vi "Filtri acquisizioni in tabella prove NEW.vi"(11 "LINGUA":i32) -> ()   [LabVIEW 2019]
uses:
  Global percorso impostazioni.vi
  <vilib>/Utility/file.llb/Write Delimited Spreadsheet (string).vi
  <vilib>/Utility/file.llb/Read Delimited Spreadsheet (string).vi
panel:
  in  "APPLICA A TUTTE":bool
  in  "carica tabella":bool
  in  "TABELLA 2":u16(ring) items=["RES FREDDO RES METER", "RES FREDDO RESISTOMAT", "A VUOTO", "A CARICO", "TERMICA", "CMECC", "ROT BLOCC", "GENERICA", "ACQ RES TERMICA", "SCORTA 2", "SCORTA 3", "EQ.TERMICO", "COPPIA MAX", "I SPUNTO", "RES INIZ VUOTO", "RES FINE VUOTO", "RES INIZ CARICO", "RES FINE CARICO"]
  in  "TABELLA":u16(ring) items=["RES FREDDO RES METER", "RES FREDDO RESISTOMAT", "A VUOTO", "A CARICO", "TERMICA", "CMECC", "ROT BLOCC", "GENERICA", "ACQ RES TERMICA", "SCORTA 2", "SCORTA 3", "EQ.TERMICO", "COPPIA MAX", "I SPUNTO", "RES INIZ VUOTO", "RES FINE VUOTO", "RES INIZ CARICO", "RES FINE CARICO"]
  in  "ORDINE COLONNE":i32(listbox)
  in  "reinizializza":bool
  in  "Save Button":bool
  in  "stop":bool
  in  "Array":T1(array[cluster]) {"Medie RT" min=-1 max=100; "decimali" min=-1 max=5}
  in  "TIPO COLLEGAMENTO":u16(ring) items=["GRUPPO ELETTROGENO", "ALTERNATORE", "GENERICO", "MOTORE C.A.", "MOTORE EEX", "MOTORE C.C.", "POMPA", "TRASFORMATORE", "POMPA EEX"]
  # "VISIBILE?  SALVA?"
  # "seleziona\ntipo collegamento"
  # "nota: -1 sul campo \"decimali\" significa che\ni decimali della grandezza in questione\nnon vengono gestiti. Utilizzare -1 per le \ngrandezze che non sono valori numerici\nad esempio tempo[h:m:s]"
  # "CONDIZIONI OBBLIGATORIE:\n\nI seguenti campi:\n\n-Banco\n-Anno\n-Numero\n-N°tabella\n-Misura\n-Tipo prova\n-Progressivo Acq\n\ndevono avere decimali=0 ed\nessere salvati per tutte le prove\n\ni campI TESTO come\n\n-tempo[h:m:s]\n-Descrizione\n...\n\ndevono avere decimali=-1"
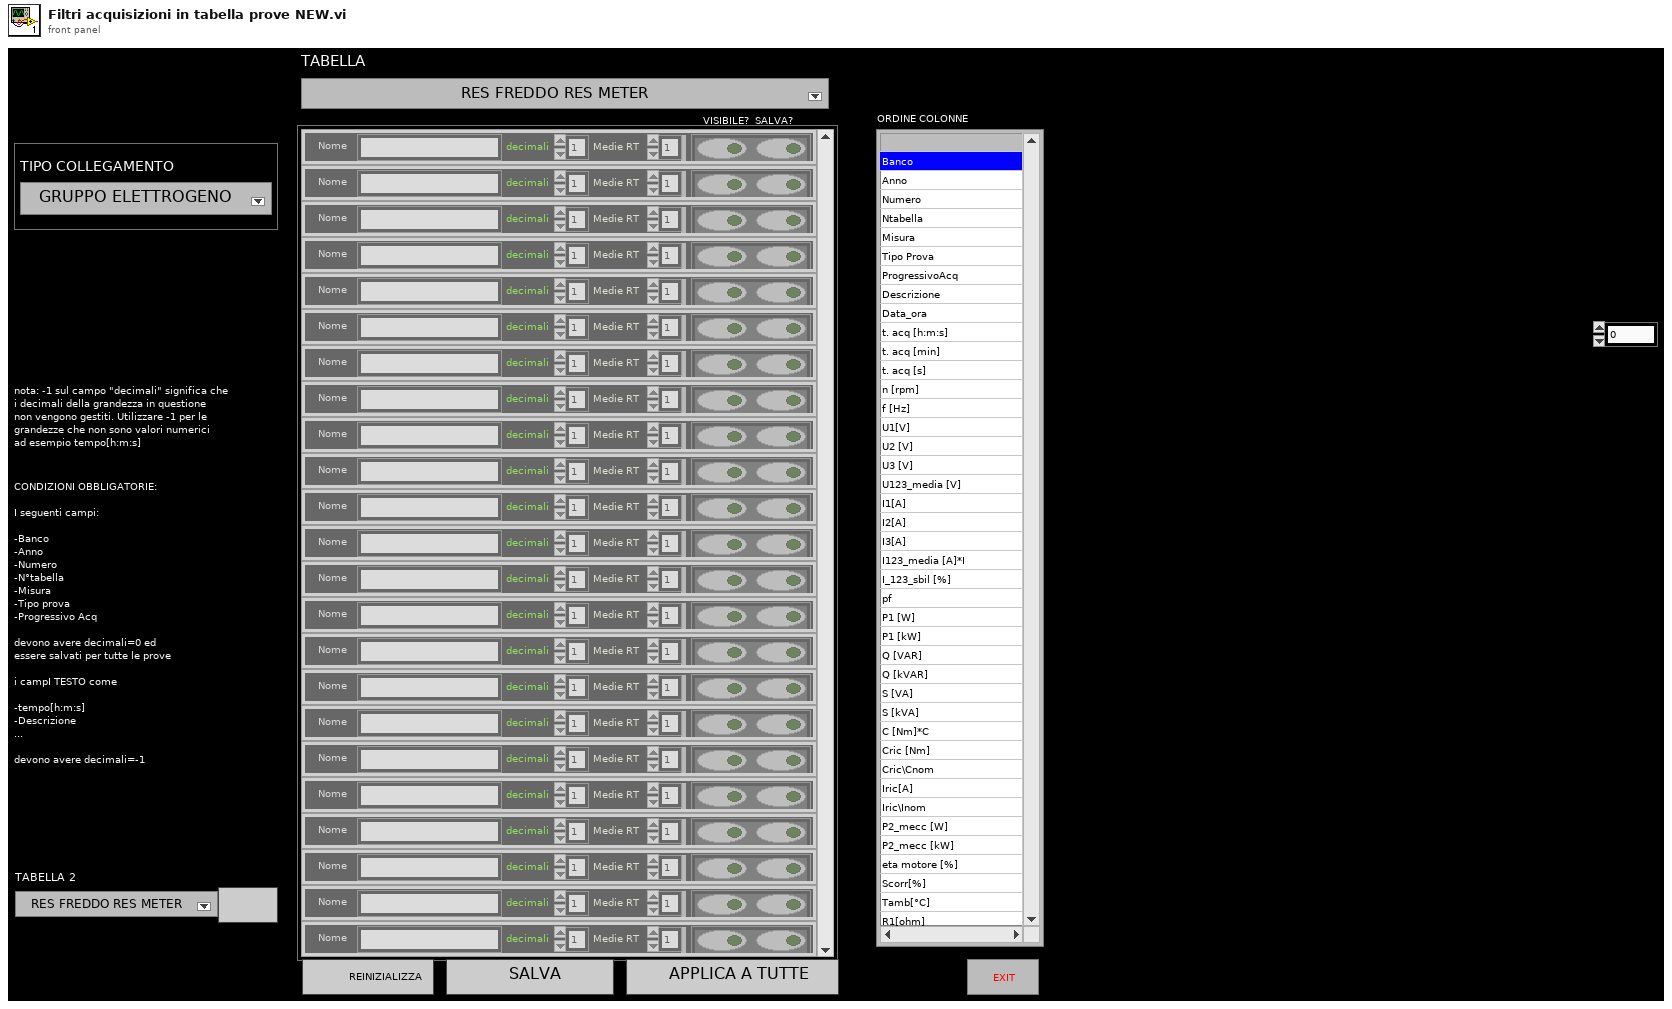
[diagram p1: front panel]
types:
  T1 = cluster{"Nome":string, "TAB":cluster{"Visibile ?":bool, "Salva?":bool}, "decimali":i8, "Medie RT":i8}[]
  T2 = cluster{"Nome":string, "TAB":cluster{"Visibile ?":bool, "Salva?":bool}, "decimali":i8, "Medie RT":i8}
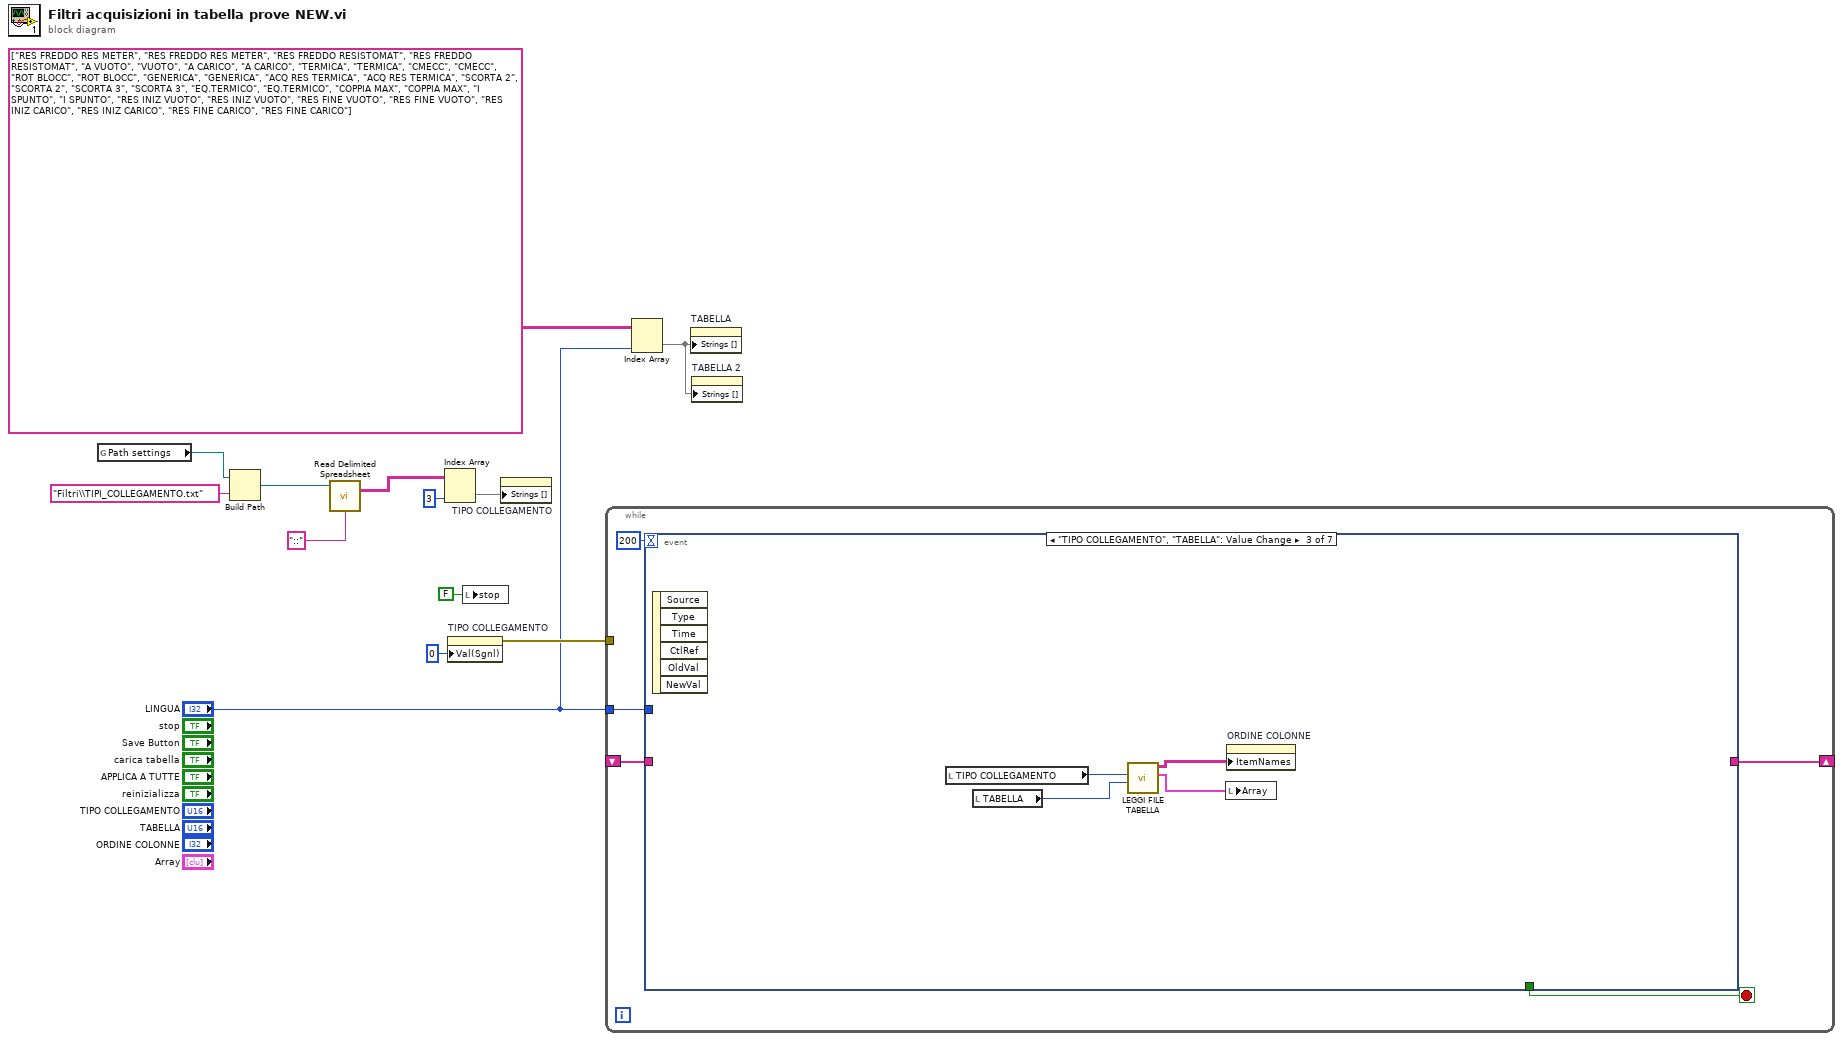
[diagram p0: block diagram]
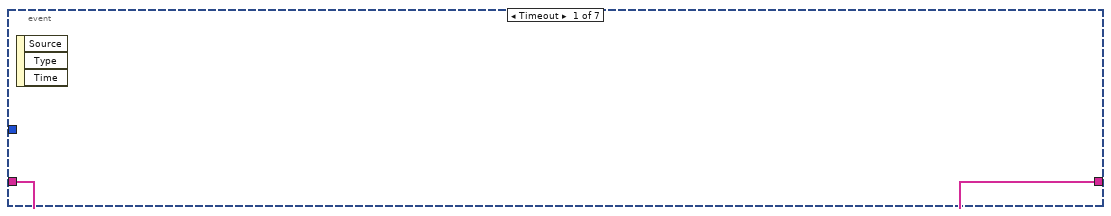
[diagram p2: hidden frame]
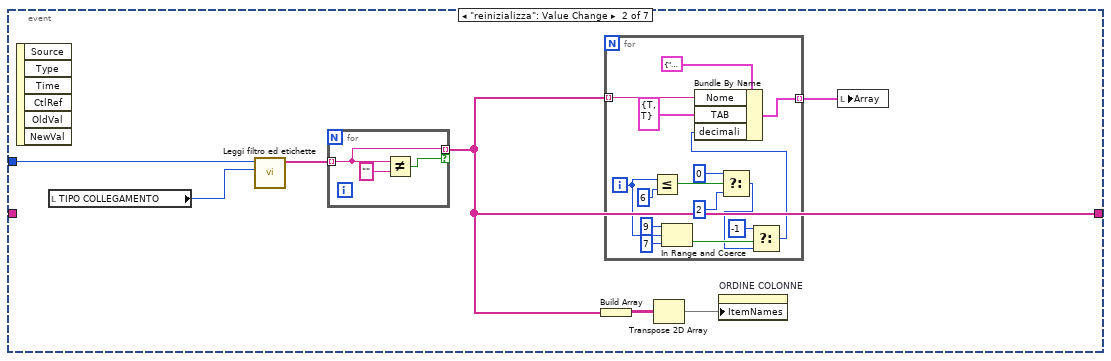
[diagram p3: hidden frame]
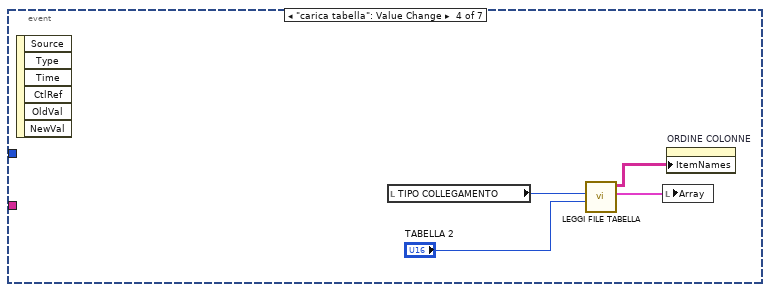
[diagram p4: hidden frame]
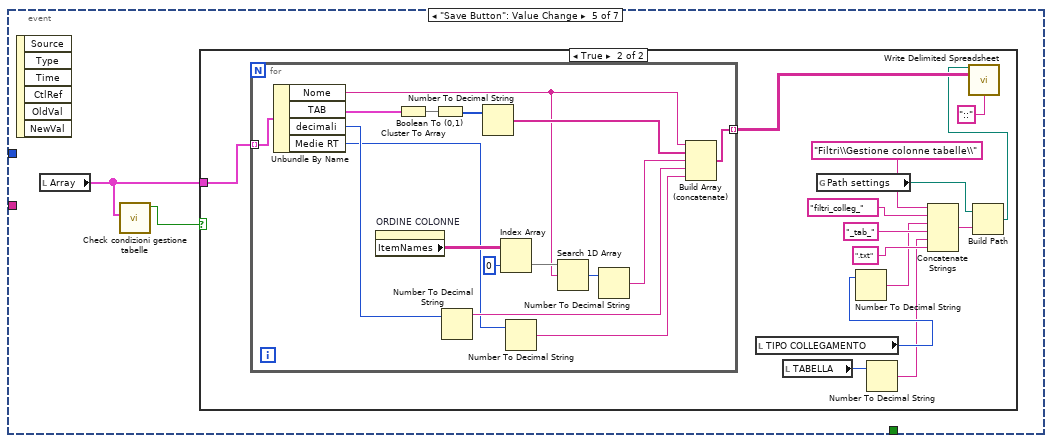
[diagram p5: hidden frame]
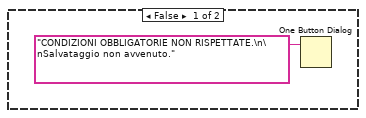
[diagram p6: hidden frame]
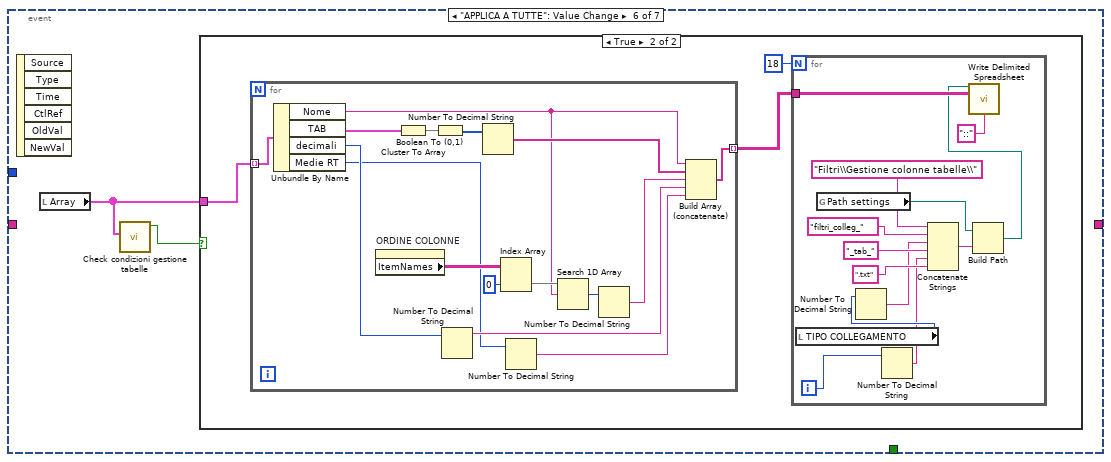
[diagram p7: hidden frame]
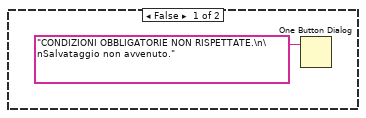
[diagram p8: hidden frame]
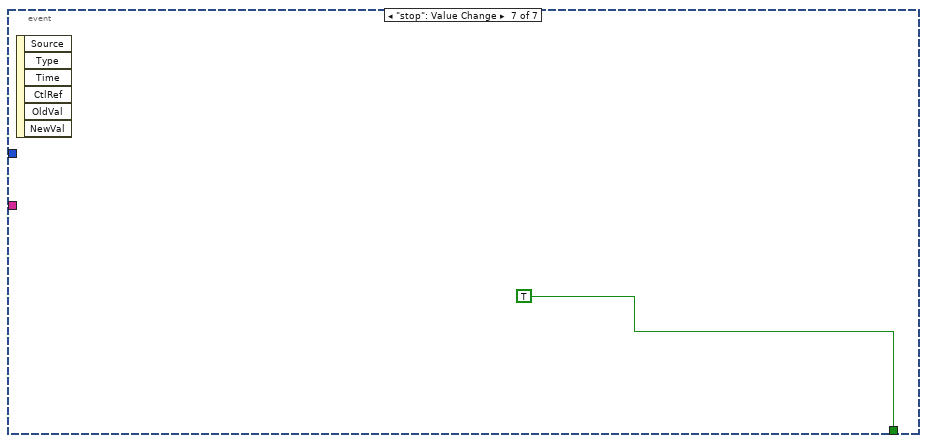
[diagram p9: hidden frame]
diagram:
  n1 = global read "Global percorso impostazioni.vi" "Path settings"() -> (w8:path)
  n2 = Build Path(base path=w8, name or relative path="Filtri\\TIPI_COLLEGAMENTO.txt") -> (appended path=w7:path)
  n3 = call-poly <vilib>:"Read Delimited Spreadsheet.vi"("file path (dialog if empty)"=w7, "delimiter (\\t)"="::" ("delimiter (\\t)")) -> ("all rows"=w5:string[][])  [unwired: 8 in, 5 out]
  n4 = Index Array(array=w5, index (col)=3 ("disabled index (col)")) -> (element=w3:string[])  [unwired: 1 in]
  n5 = property on="TIPO COLLEGAMENTO" class="Ring (strict)"("Val(Sgnl)"=u16 0 ("Value (Signaling)")) -> (error out=w11:errorcluster)  [unwired: 2 in, 1 out]
  n6 = local write "stop"(FALSE ("stop")) -> ()
  n7 = property on="TIPO COLLEGAMENTO" class="Ring (strict)"("Strings []"=w3) -> ()  [unwired: 2 in, 2 out]
  n8 = while {
    shift-right: [w18] -> _
    shift-left: _ -> [w17]
    tunnel: w11 -> [_]
    tunnel: "LINGUA" -> [w14]
    stop <- w16 stop-if-true
    n9 = event shown="[2] \"TIPO COLLEGAMENTO\", \"TABELLA\": Value Change" {
      selector: _ -> [_ _ _ _ _ _ _]
      dyn-events: _ -> [_ _ _ _ _ _ _]
      timeout: 200 -> [_ _ _ _ _ _ _]
      tunnel: [w19 w26 _ _ _ _ _] -> w18
      tunnel: w17 -> [w19 _ _ _ _ _ _]
      tunnel: [_ _ _ _ _ _ TRUE] -> w16
      tunnel: w14 -> [_ w22 _ _ _ _ _]
      event Timeout {
        n10 = event-data() -> ()  [unwired: 1 in, 3 out]
      }
      event "reinizializza": Value Change {
        n11 = event-data() -> ()  [unwired: 1 in, 6 out]
        n12 = local read "TIPO COLLEGAMENTO"() -> (w21:u16)
        n13 = call "Leggi filtro ed etichette.vi"("ID COLLEGAMENTO"=w21, "LINGUA"=w22) -> ("ETICHETTE"=w20:string[])  [unwired: 4 in, 5 out]
        n14 = for {
          tunnel: w20 -> [w43] mode=indexing
          tunnel: [w43] -> w26 mode=indexing if=w42
          n15 = Not Equal?(x=w43, y="") -> (x != y?=w42:bool)
        }
        n16 = Build Array(w26) -> (w25:string[][])
        n17 = for {
          tunnel: w26 -> [w41] mode=indexing
          tunnel: [w40] -> w23 mode=indexing
          i -> [w33]
          n18 = Less Or Equal?(x=w33, y=6) -> (x <= y?=w36:bool)
          n19 = In Range and Coerce(upper limit=9, x=w33, lower limit=7) -> (In Range?=w30:bool)  [unwired: 1 out]
          n20 = Select(t=i8 0, s=w36, f=i8 2 ("decimali")) -> (s? t:f=w28:i8)
          n21 = Select(t=i8 -1 ("decimali"), s=w30, f=w28) -> (s? t:f=w27:i8)
          n22 = Bundle By Name(cluster=T2 {"Nome"="Banco", "TAB"={"Visibile ?"=FALSE, "Salva?"=TRUE}, "decimali"=0, "Medie RT"=1} ("Cluster"), "Nome"=w41, "TAB"=cluster{"Visibile ?":bool, "Salva?":bool} {"Visibile ?"=TRUE, "Salva?"=TRUE} ("QH"), "decimali"=w27) -> (w40:T2)
        }
        n23 = Transpose 2D Array(2D array=w25) -> (transposed array=w24:string[][])
        n24 = property on="ORDINE COLONNE" class="MCListbox (strict)"("ItemNames"=w24) -> ()  [unwired: 2 in, 2 out]
        n25 = local write "Array"(w23) -> ()
      }
      event "TIPO COLLEGAMENTO", "TABELLA": Value Change {
        n26 = event-data() -> ()  [unwired: 1 in, 6 out]
        n27 = local read "TIPO COLLEGAMENTO"() -> (w48:u16)
        n28 = local read "TABELLA"() -> (w47:u16)
        n29 = call "LEGGI FILE TABELLA.vi"("INDICE TABELLA"=w47, "TIPO COLLEGAMENTO"=w48) -> ("Array"=w45:T1, "ORDINE"=w46:string[][])  [unwired: 7 in, 1 out]
        n30 = local write "Array"(w45) -> ()
        n31 = property on="ORDINE COLONNE" class="MCListbox (strict)"("ItemNames"=w46) -> ()  [unwired: 2 in, 2 out]
      }
      event "carica tabella": Value Change {
        n32 = event-data() -> ()  [unwired: 1 in, 6 out]
        n33 = local read "TIPO COLLEGAMENTO"() -> (w50:u16)
        n34 = call "LEGGI FILE TABELLA.vi"("INDICE TABELLA"="TABELLA 2", "TIPO COLLEGAMENTO"=w50) -> ("Array"=w51:T1, "ORDINE"=w52:string[][])  [unwired: 7 in, 1 out]
        n35 = local write "Array"(w51) -> ()
        n36 = property on="ORDINE COLONNE" class="MCListbox (strict)"("ItemNames"=w52) -> ()  [unwired: 2 in, 2 out]
      }
      event "Save Button": Value Change {
        n37 = event-data() -> ()  [unwired: 1 in, 6 out]
        n38 = local read "Array"() -> (w53:T1)
        n39 = call "Check condizioni gestione tabelle.vi"("Array 2"=w53) -> ("condizioni ok"=w54:bool)  [unwired: 10 in]
        n40 = case shown="True" w54 {
          tunnel: w53 -> [_ w67]
          frame False {
            n41 = One Button Dialog(message="CONDIZIONI OBBLIGATORIE NON RISPETTATE.\n\nSalvataggio non avvenuto.") -> ()  [unwired: 1 in, 1 out]
          }
          frame True {
            n42 = for {
              tunnel: w67 -> [w85] mode=indexing
              tunnel: [w84] -> w69 mode=indexing
              n43 = Unbundle By Name(w85) -> ("Nome"=w76:string, "TAB"=w83:cluster{"Visibile ?":bool, "Salva?":bool}, "decimali"=w73:i8, "Medie RT"=w70:i8)
              n44 = property on="ORDINE COLONNE" class="MCListbox (strict)"() -> ("ItemNames"=w79:string[][])  [unwired: 2 in, 2 out]
              n45 = Cluster To Array(cluster=w83) -> (array=w82:bool[])
              n46 = Boolean To (0,1)(Boolean=w82) -> (0, 1=w81:i16[])
              n47 = Number To Decimal String(number=w73) -> (decimal integer string=w72:string)  [unwired: 1 in]
              n48 = Number To Decimal String(number=w81) -> (decimal integer string=w80:string[])  [unwired: 1 in]
              n49 = Index Array(array=w79, index (col)=0 ("disabled index (col)")) -> (element=w78:string[])  [unwired: 1 in]
              n50 = Number To Decimal String(number=w70) -> (decimal integer string=w71:string)  [unwired: 1 in]
              n51 = Search 1D Array(1D array=w78, element=w76) -> (index of element=w75:i32)  [unwired: 1 in]
              n52 = Number To Decimal String(number=w75) -> (decimal integer string=w74:string)  [unwired: 1 in]
              n53 = Build Array (concatenate)(w76, w80, w74, w72, w71) -> (w84:string[])
            }
            n54 = local read "TIPO COLLEGAMENTO"() -> (w62:u16)
            n55 = local read "TABELLA"() -> (w60:u16)
            n56 = global read "Global percorso impostazioni.vi" "Path settings"() -> (w58:path)
            n57 = Number To Decimal String(number=w62) -> (decimal integer string=w61:string)  [unwired: 1 in]
            n58 = Number To Decimal String(number=w60) -> (decimal integer string=w59:string)  [unwired: 1 in]
            n59 = Concatenate Strings("Filtri\\Gestione colonne tabelle\\" ("name or relative path"), "filtri_colleg_" ("string"), w61, "_tab_" ("string"), w59, ".txt" ("string")) -> (w57:string)
            n60 = Build Path(base path=w58, name or relative path=w57) -> (appended path=w56:path)
            n61 = call-poly <vilib>:"Write Delimited Spreadsheet.vi"("file path (dialog if empty)"=w56, "2D data"=w69, "delimiter (\\t)"="::" ("delimiter (\\t)")) -> ()  [unwired: 11 in, 2 out]
          }
        }
      }
      event "APPLICA A TUTTE": Value Change {
        n62 = event-data() -> ()  [unwired: 1 in, 6 out]
        n63 = local read "Array"() -> (w86:T1)
        n64 = call "Check condizioni gestione tabelle.vi"("Array 2"=w86) -> ("condizioni ok"=w87:bool)  [unwired: 10 in]
        n65 = case shown="True" w87 {
          tunnel: w86 -> [_ w90]
          frame False {
            n66 = One Button Dialog(message="CONDIZIONI OBBLIGATORIE NON RISPETTATE.\n\nSalvataggio non avvenuto.") -> ()  [unwired: 1 in, 1 out]
          }
          frame True {
            n67 = for {
              tunnel: w90 -> [w120] mode=indexing
              tunnel: [w119] -> w91 mode=indexing
              n68 = Unbundle By Name(w120) -> ("Nome"=w111:string, "TAB"=w118:cluster{"Visibile ?":bool, "Salva?":bool}, "decimali"=w108:i8, "Medie RT"=w105:i8)
              n69 = property on="ORDINE COLONNE" class="MCListbox (strict)"() -> ("ItemNames"=w114:string[][])  [unwired: 2 in, 2 out]
              n70 = Cluster To Array(cluster=w118) -> (array=w117:bool[])
              n71 = Boolean To (0,1)(Boolean=w117) -> (0, 1=w116:i16[])
              n72 = Number To Decimal String(number=w108) -> (decimal integer string=w107:string)  [unwired: 1 in]
              n73 = Number To Decimal String(number=w116) -> (decimal integer string=w115:string[])  [unwired: 1 in]
              n74 = Index Array(array=w114, index (col)=0 ("disabled index (col)")) -> (element=w113:string[])  [unwired: 1 in]
              n75 = Number To Decimal String(number=w105) -> (decimal integer string=w106:string)  [unwired: 1 in]
              n76 = Search 1D Array(1D array=w113, element=w111) -> (index of element=w110:i32)  [unwired: 1 in]
              n77 = Number To Decimal String(number=w110) -> (decimal integer string=w109:string)  [unwired: 1 in]
              n78 = Build Array (concatenate)(w111, w115, w109, w107, w106) -> (w119:string[])
            }
            n79 = for {
              N: 18 -> [_]
              tunnel: w91 -> [w104]
              i -> [w92]
              n80 = local read "TIPO COLLEGAMENTO"() -> (w98:u16)
              n81 = global read "Global percorso impostazioni.vi" "Path settings"() -> (w95:path)
              n82 = Number To Decimal String(number=w98) -> (decimal integer string=w97:string)  [unwired: 1 in]
              n83 = Number To Decimal String(number=w92) -> (decimal integer string=w96:string)  [unwired: 1 in]
              n84 = Concatenate Strings("Filtri\\Gestione colonne tabelle\\" ("name or relative path"), "filtri_colleg_" ("string"), w97, "_tab_" ("string"), w96, ".txt" ("string")) -> (w94:string)
              n85 = Build Path(base path=w95, name or relative path=w94) -> (appended path=w93:path)
              n86 = call-poly <vilib>:"Write Delimited Spreadsheet.vi"("file path (dialog if empty)"=w93, "2D data"=w104, "delimiter (\\t)"="::" ("delimiter (\\t)")) -> ()  [unwired: 11 in, 2 out]
            }
          }
        }
      }
      event "stop": Value Change {
        n87 = event-data() -> ()  [unwired: 1 in, 6 out]
      }
    }
  }
  n88 = Index Array(array=string[][] [["RES FREDDO RES METER", "RES FREDDO RES METER"], ["RES FREDDO RESISTOMAT", "RES FREDDO RESISTOMAT"], ["A VUOTO", "VUOTO"], ["A CARICO", "A CARICO"], ["TERMICA", "TERMICA"], ["CMECC", "CMECC"], ["ROT BLOCC", "ROT BLOCC"], ["GENERICA", "GENERICA"], ["ACQ RES TERMICA", "ACQ RES TERMICA"], ["SCORTA 2", "SCORTA 2"], ["SCORTA 3", "SCORTA 3"], ["EQ.TERMICO", "EQ.TERMICO"], ["COPPIA MAX", "COPPIA MAX"], ["I SPUNTO", "I SPUNTO"], ["RES INIZ VUOTO", "RES INIZ VUOTO"], ["RES FINE VUOTO", "RES FINE VUOTO"], ["RES INIZ CARICO", "RES INIZ CARICO"], ["RES FINE CARICO", "RES FINE CARICO"]], index (col)="LINGUA") -> (element=w1:string[])  [unwired: 1 in]
  n89 = property on="TABELLA" class="Ring (strict)"("Strings []"=w1) -> ()  [unwired: 2 in, 2 out]
  n90 = property on="TABELLA 2" class="Ring (strict)"("Strings []"=w1) -> ()  [unwired: 2 in, 2 out]
